vi "Check Log (SubVI).vi"(8 "error in (no error)":errorcluster, 11 "Intrinsic Data Cluster TD in":T1) -> (0 "error out":errorcluster, 3 "Intrinsic Data Cluster TD out":T1)   [LabVIEW 2016]
uses:
  Intrinsic data TD.ctl
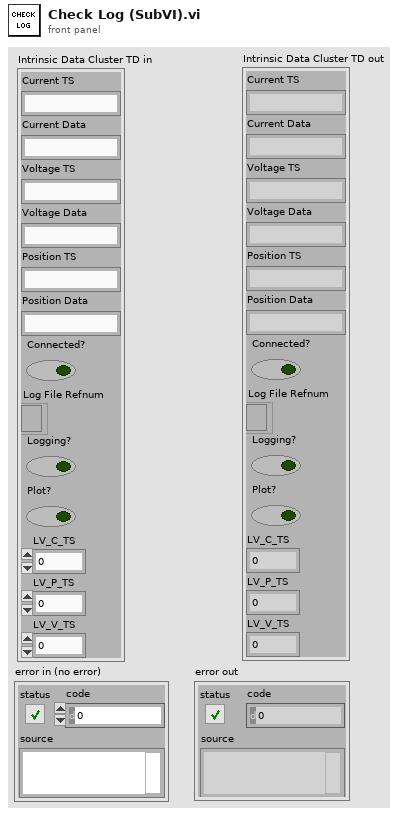
[diagram p1: front panel]
types:
  T1 = typedef "Intrinsic data TD.ctl" = cluster{"Current TS":string, "Current Data":string, "Voltage TS":string, "Voltage Data":string, "Position TS":string, "Position Data":string, "Connected?":bool, "Log File Refnum":refnum<file>, "Logging?":bool, "Plot?":bool, "LV_C_TS":dbl, "LV_P_TS":dbl, "LV_V_TS":dbl}
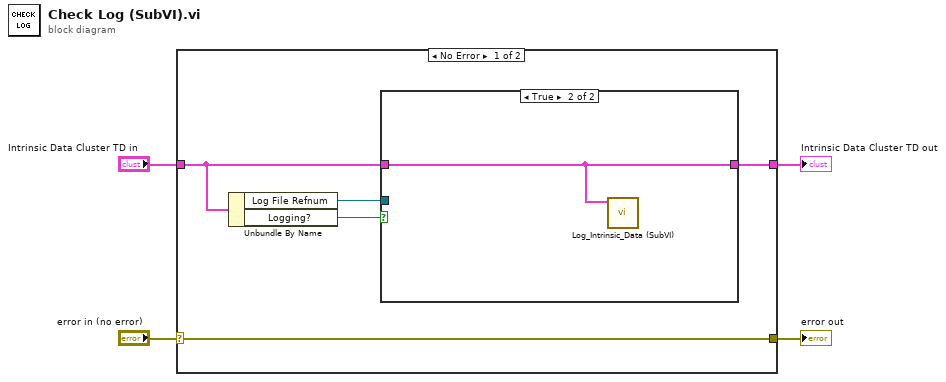
[diagram p0: block diagram]
diagram:
  n1 = case shown="No Error" "error in (no error)" {
    selector: "error in (no error)" -> [w5 w12]
    tunnel: [w9 w13] -> w4
    tunnel: "Intrinsic Data Cluster TD in" -> [w8 w13]
    tunnel: [w5 w12] -> w1
    frame No Error {
      n2 = Unbundle By Name(w8) -> ("Log File Refnum"=w7:refnum<file>, "Logging?"=w6:bool)
      n3 = case shown="True" w6 {
        tunnel: w7 -> [_ _]
        tunnel: w8 -> [w10 w11]
        tunnel: [w10 w11] -> w9
        frame False {
        }
        frame True {
          n4 = call "Log_Intrinsic_Data (SubVI).vi"("Intrinsic Data Cluster TD in"=w11) -> ()  [unwired: 10 in, 1 out]
        }
      }
    }
    frame Error {
    }
  }
  "Intrinsic Data Cluster TD out" <- w4
  "error out" <- w1
